vi "Import Resources From File.vi"(8 "error in (no error)":errorcluster, 10 "file path (use dialog)":path, 11 "LangFile.lvclass in":refnum<class "Resource Data.lvclass">) -> (0 "error out":errorcluster, 3 "LangFile.lvclass out":refnum<class "Resource Data.lvclass">)   [LabVIEW 2013, in "SET Project Data.lvlib" / "Resource Data.lvclass"]
uses:
  Resource Data.lvclass
  Types/ProjFile_Resource Entry.ctl
  SET Project Data.lvlib
  Lib/Robust CSV/SET_Robust CSV (UTF-16).lvlib
  Lib/Unicode/SET_Unicode Tools.lvlib
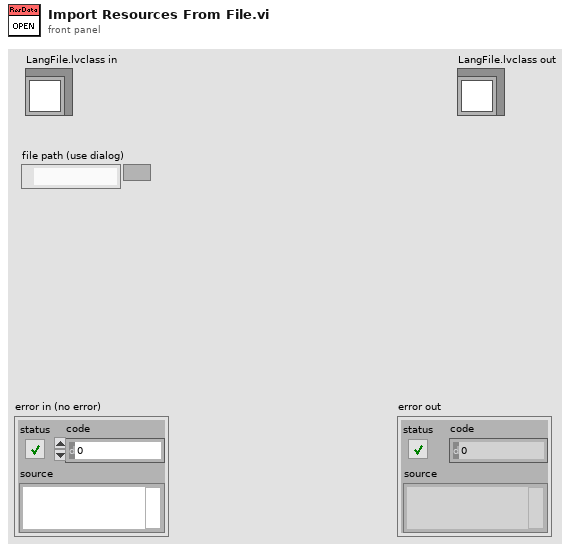
[diagram p1: front panel]
types:
  T1 = typedef "SET Project Data.lvlib/ProjFile_Resource Entry.ctl" = cluster{"RID":string, "Tag":string, "Strings [] (UTF-16)":string[], "Shared?":bool}
  T2 = typedef "SET Project Data.lvlib/ProjFile_Language Entry.ctl" = cluster{"Tag":string, "Name":string, "Code Page":u16}
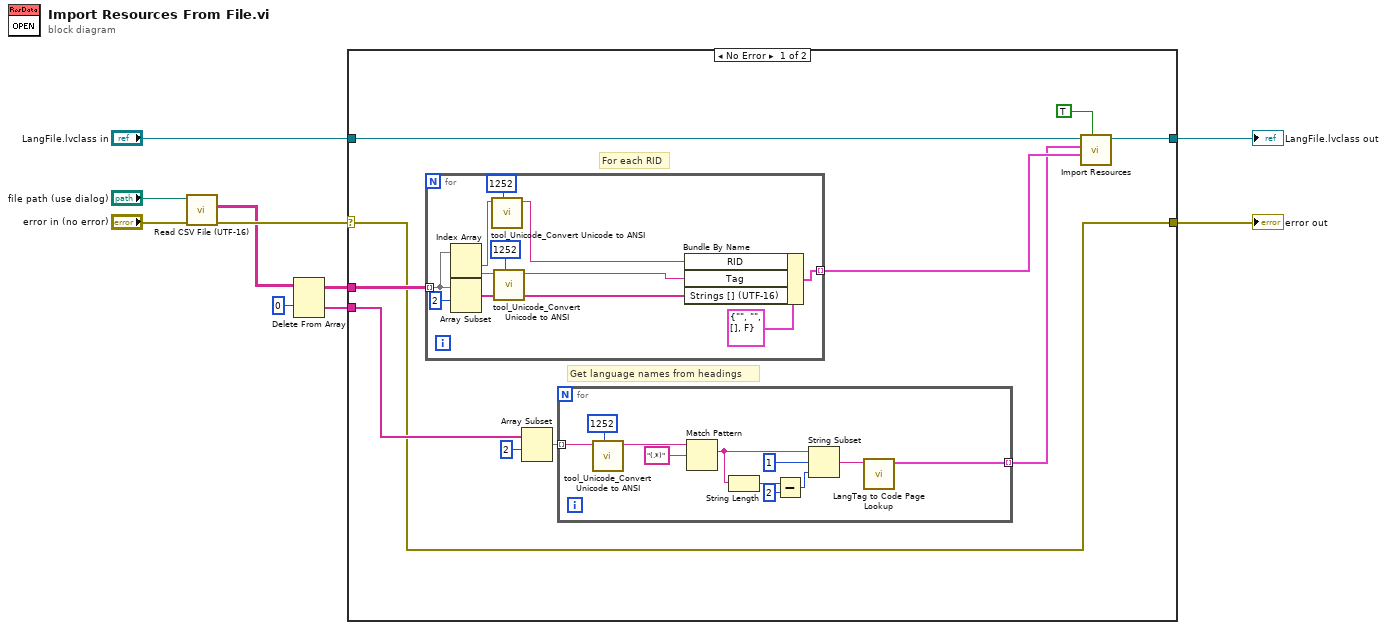
[diagram p0: block diagram]
diagram:
  n1 = call "Read CSV File (UTF-16).vi"("error in (no error)"="error in (no error)", "file path in"="file path (use dialog)") -> ("error out"=w5:errorcluster, "2-D array *UTF-16"=w4:string[][])  [unwired: 7 in, 1 out]
  n2 = Delete From Array(array=w4, index (row)=0) -> (deleted portion=w1:string[], array with subset deleted=w2:string[][])  [unwired: 2 in]
  n3 = case shown="No Error" w5 {
    selector: w5 -> [w12 w44]
    tunnel: [w12 w44] -> w10
    tunnel: "LangFile.lvclass in" -> [w16 w43]
    tunnel: [w14 w43] -> w9
    tunnel: w1 -> [w18 _]
    tunnel: w2 -> [w17 _]
    frame No Error {
      # "For each RID"
      # "Get language names from headings"
      n4 = for {
        tunnel: [w39] -> w15 mode=indexing
        tunnel: w17 -> [w38] mode=indexing
        n5 = Index Array(array=w38) -> (element #1=w35:string, element #2=w37:string)  [unwired: 2 in]
        n6 = Array Subset(array=w38, index=2) -> (w40:string[])  [unwired: 1 in]
        n7 = call "tool_Unicode_Convert Unicode to ANSI.vi"("Dest. Code Page"=u16 1252, "WideChar (UTF16-LE)"=w35) -> ("MultiByteStr (ANSI)"=w32:string)  [unwired: 8 in, 1 out]
        n8 = call "tool_Unicode_Convert Unicode to ANSI.vi"("Dest. Code Page"=u16 1252, "WideChar (UTF16-LE)"=w37) -> ("MultiByteStr (ANSI)"=w36:string)  [unwired: 8 in, 1 out]
        n9 = Bundle By Name(cluster=T1 {"RID"="", "Tag"="", "Strings [] (UTF-16)"=[], "Shared?"=FALSE} ("Resource"), "RID"=w32, "Tag"=w36, "Strings [] (UTF-16)"=w40) -> (w39:T1)
      }
      n10 = Array Subset(array=w18, index=2) -> (w19:string[])  [unwired: 1 in]
      n11 = for {
        tunnel: w19 -> [w24] mode=indexing
        tunnel: [w21] -> w11 mode=indexing
        n12 = call "tool_Unicode_Convert Unicode to ANSI.vi"("Dest. Code Page"=u16 1252, "WideChar (UTF16-LE)"=w24) -> ("MultiByteStr (ANSI)"=w23:string)  [unwired: 8 in, 1 out]
        n13 = Match Pattern(string=w23, regular expression="(.*)") -> (match substring=w29:string)  [unwired: 1 in, 3 out]
        n14 = String Length(string=w29) -> (length=w28:i32)
        n15 = Subtract(x=w28, y=2) -> (x-y=w26:i32)
        n16 = String Subset(string=w29, offset (0)=1, length (rest)=w26) -> (substring=w25:string)
        n17 = call "LangTag to Code Page Lookup.vi"("Tag"=w25) -> ("Language"=w21:T2)  [unwired: 9 in, 1 out]
      }
      n18 = call "Import Resources.vi"("Ignore New? (F)"=TRUE, "Resources []"=w15, "Languages []"=w11, "LangFile.lvclass in"=w16) -> ("LangFile.lvclass out"=w14:refnum<class "Resource Data.lvclass">)  [unwired: 7 in]
    }
    frame Error {
    }
  }
  "error out" <- w10
  "LangFile.lvclass out" <- w9
